vi "CaseBasedLED.vi"() -> ()   [LabVIEW 2021]
uses:
  LEDStates.ctl
  <vilib>/MakerHub/LINX/Public/Peripherals/Digital/Digital Write 1 Chan.vi
  <vilib>/MakerHub/LINX/Public/Peripherals/Digital/Digital Write N Chans.vi
  <vilib>/MakerHub/LINX/Private/Local IO/LinxDigitalWrite.vi
  <vilib>/MakerHub/LINX/Public/Utilities/Check Channel.vi
  <vilib>/MakerHub/LINX/Public/Utilities/Open Serial.vi
  <vilib>/MakerHub/LINX/Private/Utilties/Generate Error.vi
  <vilib>/MakerHub/LINX/LMH-LINX.lvlib
panel:
  out "Indicator":bool
  in  "DO Channel":u8
  in  "Serial Port":refnum<visa-resource-name>="N/A"
  in  "Switch 1":bool
  in  "Switch 2":bool
  in  "Stop":bool
  in  "Pause":bool
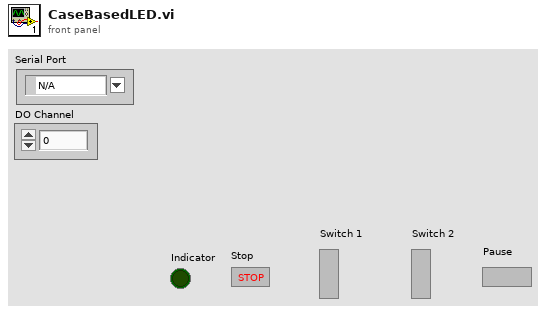
[diagram p1: front panel]
types:
  T1 = typedef "LEDStates.ctl" = enum16{"Play", "Pause"}
  T2 = typedef "LMH-LINX.lvlib/LINX Ref.ctl" = cluster{"IO":T3, "Interface":T4, "LINX Device Config":T5}
  T3 = typedef "LMH-LINX.lvlib/Platform.ctl" = enum16{"Remote", "Local"}
  T4 = typedef "LMH-LINX.lvlib/Interface.ctl" = enum16{"Serial", "TCP"}
  T5 = typedef "LMH-LINX.lvlib/Device.lvlib/LINX Device Config.ctl" = cluster{"Interface":T4, "COM Port":refnum<visa-resource-name>, "TCP Configuration":T6, "Device Family":u8, "Device ID":u8, "Device Name":string, "TCP Ref":refnum<k5>, "Channels":T7}
  T6 = typedef "LMH-LINX.lvlib/Device.lvlib/TCP Config.ctl" = cluster{"IP Address":string, "Port":u16}
  T7 = typedef "LMH-LINX.lvlib/Channels.ctl" = cluster{"DI":u8[], "DO":u8[], "AI":u8[], "AO":u8[], "PWM":u8[], "QE":u8[], "UART":u8[], "I2C 2":u8[], "SPI":u8[], "CAN":u8[], "Servo":u8[], "AI Ref (V)":dbl, "AI Resolution (Bits)":u8, "AO Ref (V)":dbl, "AO Resolution (Bits)":u8}
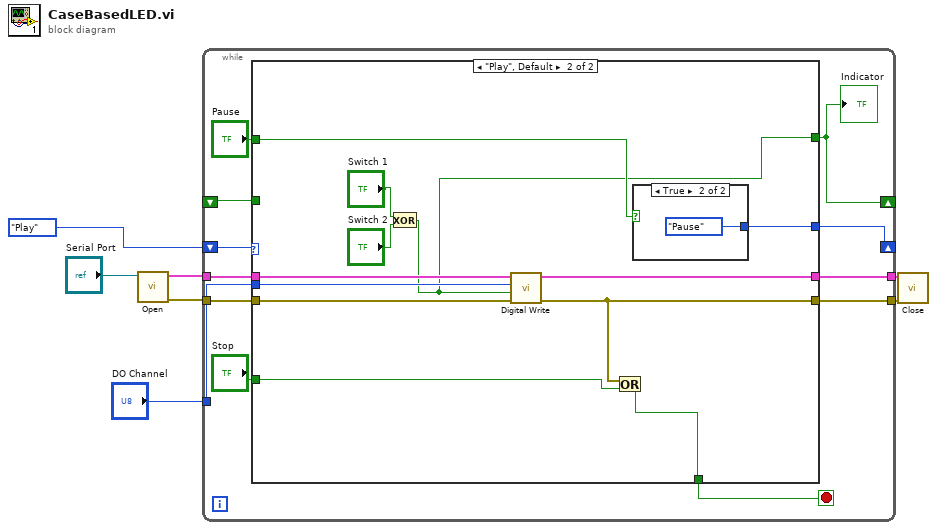
[diagram p0: block diagram]
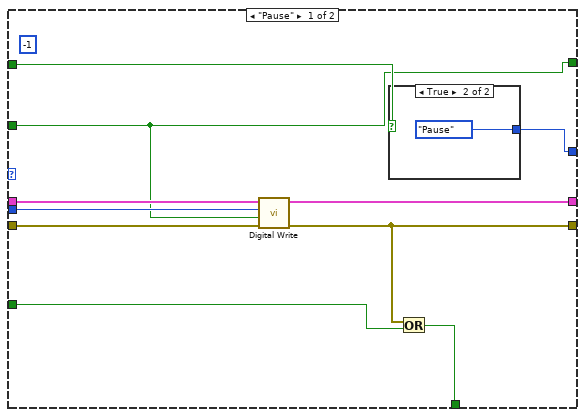
[diagram p2: hidden frame]
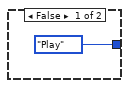
[diagram p3: hidden frame]
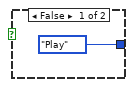
[diagram p4: hidden frame]
diagram:
  n1 = call-poly <vilib>:"Open.vi"("Serial Port"="Serial Port") -> ("Error Out"=w5:errorcluster, "LINX Resource"=w7:T2)  [unwired: 8 in, 1 out]
  n2 = while {
    tunnel: w7 -> [w19]
    tunnel: [w10] -> w6
    tunnel: w5 -> [w18]
    tunnel: [w16] -> w4
    tunnel: "DO Channel" -> [w17]
    shift-right: [w14] -> _
    shift-left: LEDStates."Play" ("States") -> [w13]
    shift-right: [w8] -> _
    shift-left: _ -> [w9]
    stop <- w15 stop-if-true
    n3 = case shown="\"Play\", Default" w13 {
      tunnel: w19 -> [w25 w43]
      tunnel: w18 -> [w23 w41]
      tunnel: w17 -> [w21 w40]
      tunnel: [w22 w39] -> w16
      tunnel: [w29 w38] -> w15
      tunnel: [w28 w37] -> w14
      tunnel: "Pause" -> [w27 w36]
      tunnel: "Stop" -> [w26 w35]
      tunnel: [w24 w42] -> w10
      tunnel: [w20 w32] -> w8
      tunnel: w9 -> [w20 _]
      frame "Pause" {
        (unwired) -1
        n4 = call-poly <vilib>:"Digital Write.vi"("Error In"=w23, "Output Value"=w20, "DO Channel"=w21, "LINX Resource"=w25) -> ("Error Out"=w22:errorcluster, "LINX Resource"=w24:T2)  [unwired: 6 in]
        n5 = case shown="True" w27 {
          tunnel: [LEDStates."Play" ("States") LEDStates."Pause" ("States")] -> w28
          frame False {
          }
          frame True {
          }
        }
        n6 = Or(x=w22, y=w26) -> (x .or. y?=w29:bool)
      }
      frame "Play", Default {
        n7 = Exclusive Or(1:"Switch 2", 2:"Switch 1") -> (0:w32:bool)
        n8 = call-poly <vilib>:"Digital Write.vi"("Error In"=w41, "Output Value"=w32, "DO Channel"=w40, "LINX Resource"=w43) -> ("Error Out"=w39:errorcluster, "LINX Resource"=w42:T2)  [unwired: 6 in]
        n9 = Or(x=w39, y=w35) -> (x .or. y?=w38:bool)
        n10 = case shown="True" w36 {
          tunnel: [LEDStates."Play" ("States") LEDStates."Pause" ("States")] -> w37
          frame False {
          }
          frame True {
          }
        }
      }
    }
    "Indicator" <- w8
  }
  n11 = call <vilib>:"Close.vi"("Error In"=w4, "LINX Resource"=w6) -> ()  [unwired: 9 in, 1 out]
